vi "setUp.vi"(8 "error in (no error)":errorcluster, 11 "Unit Tests for Runner in":refnum<class "Unit Tests for Runner.lvclass">) -> (0 "error out":errorcluster, 3 "Unit Tests for Runner out":refnum<class "Unit Tests for Runner.lvclass">)   [LabVIEW 2013, in "Unit Tests for Runner.lvclass"]
uses:
  Unit Tests for Runner.lvclass
  Unit Tests for Runner.lvclass/Unit Tests for Runner.ctl
  classes/Test Runner/Test Runner.lvclass
  support files/root define test.vi
  support files/lone test.vi
  classes/Test/Test.lvclass
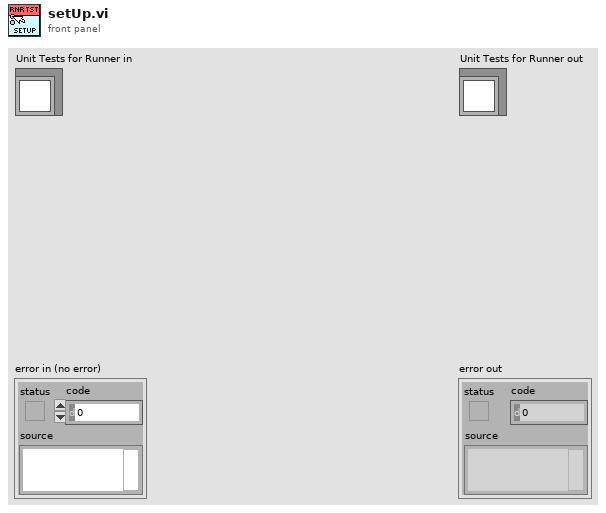
[diagram p1: front panel]
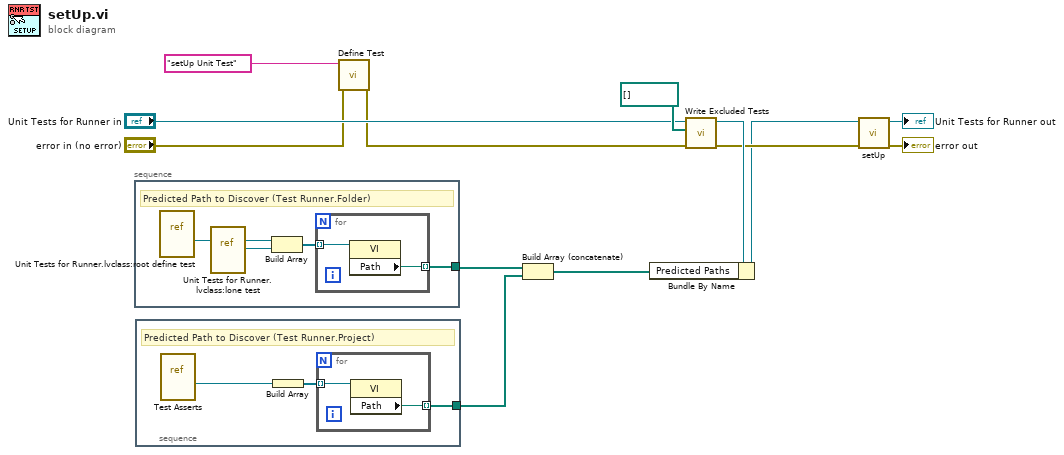
[diagram p0: block diagram]
diagram:
  n1 = stacked-sequence {
    tunnel: [w14] -> w8
    frame #0 {
      # "Predicted Path to Discover (Test Runner.Folder)"
      n2 = vi-ref "Unit Tests for Runner.lvclass:root define test.vi"() -> (w17:refnum<vi>)
      n3 = vi-ref "Unit Tests for Runner.lvclass:lone test.vi"() -> (w16:refnum<vi>)
      n4 = Build Array(w17, w16) -> (w15:refnum<vi>[])
      n5 = for {
        tunnel: w15 -> [w19] mode=indexing
        tunnel: [w18] -> w14 mode=indexing
        n6 = property on="Property Node" class="VI"(reference=w19) -> ("Path"=w18:path)  [unwired: 1 in, 2 out]
      }
    }
  }
  n7 = stacked-sequence {
    tunnel: [w20] -> w7
    frame #0 {
      # "Predicted Path to Discover (Test Runner.Project)"
      n8 = vi-ref "Test Asserts.vi"() -> (w22:refnum<vi>)
      n9 = Build Array(w22) -> (w21:refnum<vi>[])
      n10 = for {
        tunnel: w21 -> [w24] mode=indexing
        tunnel: [w23] -> w20 mode=indexing
        n11 = property on="Property Node" class="VI"(reference=w24) -> ("Path"=w23:path)  [unwired: 1 in, 2 out]
      }
    }
  }
  n12 = call "Define Test.vi"("error in (no error)"="error in (no error)", "Label (VI Title)"="setUp Unit Test") -> ("error out"=w1:errorcluster)  [unwired: 9 in]
  n13 = Build Array (concatenate)(w8, w7) -> (w6:path[])
  n14 = call "Write Excluded Tests.vi"("error in (no error)"=w1, "Excluded Tests"=path[] [], "Test Runner in"="Unit Tests for Runner in") -> ("error out"=w5:errorcluster, "Test Runner out"=w10:refnum<class "Unit Tests for Runner.lvclass">)  [unwired: 7 in]
  n15 = Bundle By Name(cluster=w10, "Predicted Paths"=w6) -> (w4:refnum<class "Unit Tests for Runner.lvclass">)
  n16 = call-parent "setUp.vi"("error in (no error)"=w5, "Test Runner in"=w4) -> ("error out"=→"error out":errorcluster, "Test Runner out"=→"Unit Tests for Runner out":refnum<class "Unit Tests for Runner.lvclass">)  [unwired: 8 in]
